vi "File.Open.vi"(8 "error in":errorcluster, 11 "file":path) -> (0 "error out":errorcluster, 3 "File ref out":refnum<file>)   [LabVIEW 2016]
doc: "Writes to a file.\nIf <B>append</B> is false (default), the file will be rewritten.\nIf <B>append</B> is true, the new data will be appended to the file.\nSupports a <B>header</B> line which will be placed on top of the file when it is created or rewritten. This <B>header</B> line requires a newline at the end."
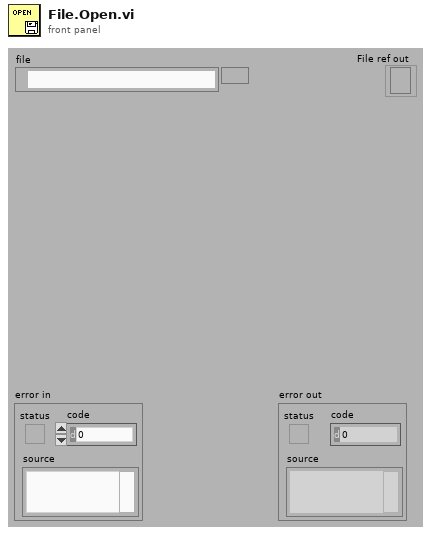
[diagram p1: front panel]
types:
  T1 = enum16{"open", "replace", "create", "open or create", "replace or create", "replace or create with confirmation"}
  T2 = enum16{"deny read/write", "deny write-only", "deny none"}
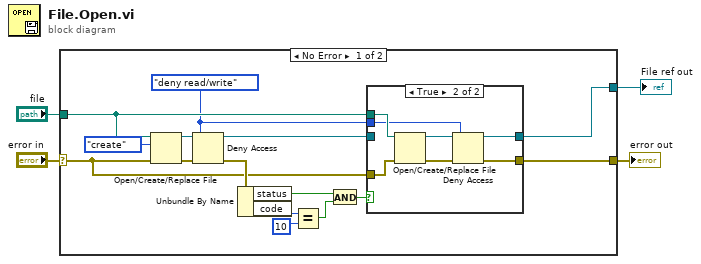
[diagram p0: block diagram]
diagram:
  n1 = case shown="No Error" "error in" {
    selector: "error in" -> [w16 w29]
    tunnel: [w8 w29] -> w4
    tunnel: "file" -> [w19 _]
    tunnel: [w7 _] -> w1
    frame No Error {
      w6 = T2."deny read/write" ("deny mode (2)")
      n2 = Open/Create/Replace File(file path (use dialog)=w19, error in=w16, operation (0:open)=T1."create") -> (refnum out=w9:refnum<file>, error out=w10:errorcluster)  [unwired: 1 in, 3 out]
      n3 = Deny Access(4:w10, 6:w6, 7:w9) -> (0:w17:errorcluster, 3:w18:refnum<file>)
      n4 = Unbundle By Name(w17) -> ("status"=w12:bool, "code"=w15:i32)
      n5 = Equal?(x=w15, y=10) -> (x = y?=w13:bool)
      n6 = And(x=w12, y=w13) -> (x .and. y?=w11:bool)
      n7 = case shown="True" w11 {
        tunnel: [w20 w28] -> w8
        tunnel: w19 -> [_ w27]
        tunnel: w18 -> [w21 _]
        tunnel: [w21 w26] -> w7
        tunnel: w16 -> [w20 w25]
        tunnel: w6 -> [_ w22]
        frame False {
        }
        frame True {
          n8 = Open/Create/Replace File(file path (use dialog)=w27, error in=w25) -> (refnum out=w23:refnum<file>, error out=w24:errorcluster)  [unwired: 5 out]
          n9 = Deny Access(4:w24, 6:w22, 7:w23) -> (0:w28:errorcluster, 3:w26:refnum<file>)
        }
      }
    }
    frame Error {
    }
  }
  "error out" <- w4
  "File ref out" <- w1
